vi "GetSRdata.vi"(8 "Error In":errorcluster) -> (0 "Error Out":errorcluster, 3 "SRList":T1 {"SR#" format="%#_10g"})   [LabVIEW 2017, in "Server.lvlib" / "Oracle.lvlib"]
uses:
  Oracle.lvlib
  TypeDefs/SR List.ctl
  TypeDefs/SR Data.ctl
  Server.lvlib
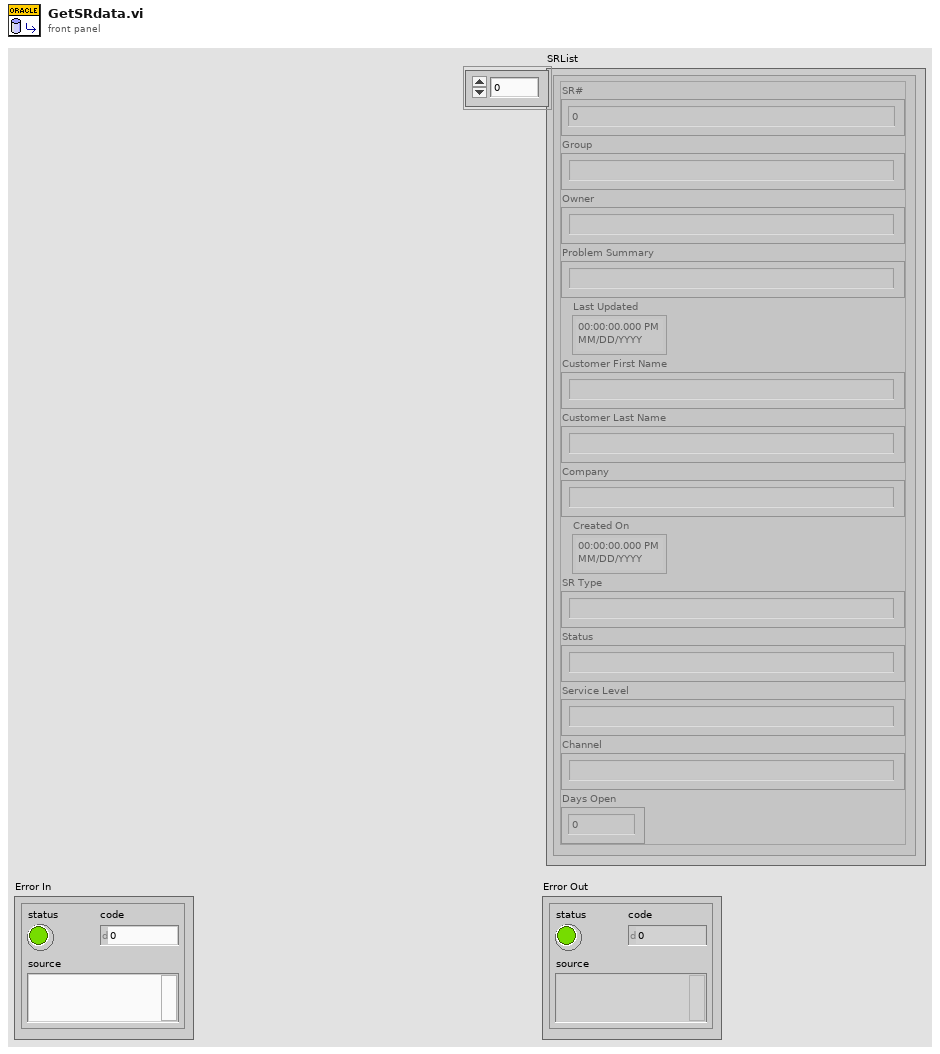
[diagram p1: front panel]
types:
  T1 = typedef "Server.lvlib/SR List.ctl" = T2[]
  T2 = typedef "Server.lvlib/SR Data.ctl" = cluster{"SR#":dbl, "Group":string, "Owner":string, "Problem Summary":string, "Last Updated":timestamp, "Customer First Name":string, "Customer Last Name":string, "Company":string, "Created On":timestamp, "SR Type":string, "Status":string, "Service Level":string, "Channel":string, "Days Open":dbl}
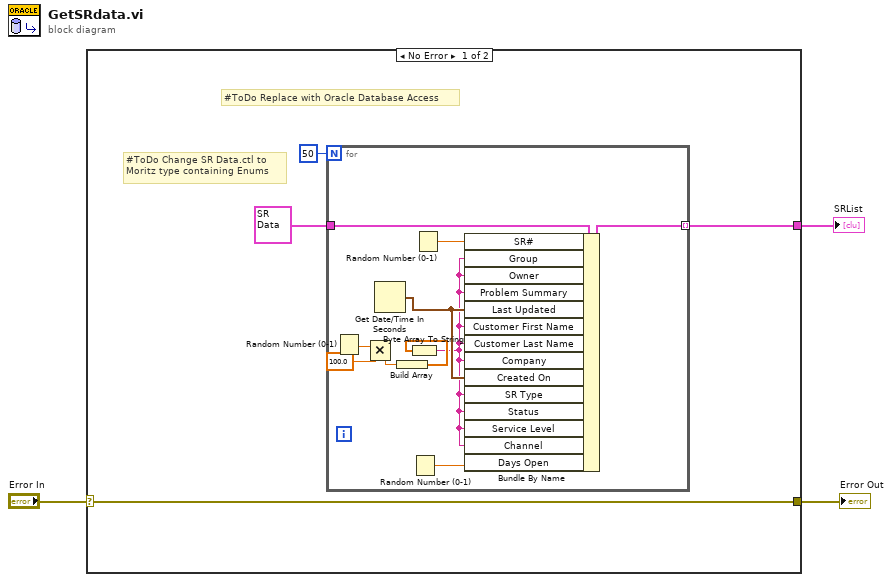
[diagram p0: block diagram]
diagram:
  n1 = case shown="No Error" "Error In" {
    selector: "Error In" -> [w7 w18]
    tunnel: [w7 w18] -> w2
    tunnel: [w5 _] -> w1
    frame No Error {
      # "#ToDo Change SR Data.ctl to\nMoritz type containing Enums"
      # "#ToDo Replace with Oracle Database Access"
      n2 = for {
        N: 50 -> [_]
        tunnel: T2 {"SR#"=0.0, "Group"="", "Owner"="", "Problem Summary"="", "Last Updated"=timestamp(0 s since 1904-01-01), "Customer First Name"="", "Customer Last Name"="", "Company"="", "Created On"=timestamp(0 s since 1904-01-01), "SR Type"="", "Status"="", "Service Level"="", "Channel"="", "Days Open"=0.0} ("SR Data") -> [w17]
        tunnel: [w16] -> w5 mode=indexing
        n3 = Random Number (0-1)() -> (number: 0 to 1=w13:dbl)
        n4 = Multiply(x=w13, y=100.0) -> (x*y=w11:dbl)
        n5 = Get Date/Time In Seconds() -> (seconds since 1Jan1904=w9:timestamp)
        n6 = Build Array(w11) -> (w10:dbl[])
        n7 = Byte Array To String(unsigned byte array=w10) -> (string=w8:string)
        n8 = Random Number (0-1)() -> (number: 0 to 1=w14:dbl)
        n9 = Random Number (0-1)() -> (number: 0 to 1=w15:dbl)
        n10 = Bundle By Name(cluster=w17, "SR#"=w15, "Group"=w8, "Owner"=w8, "Problem Summary"=w8, "Last Updated"=w9, "Customer First Name"=w8, "Customer Last Name"=w8, "Company"=w8, "Created On"=w9, "SR Type"=w8, "Status"=w8, "Service Level"=w8, "Channel"=w8, "Days Open"=w14) -> (w16:T2)
      }
    }
    frame Error {
    }
  }
  "Error Out" <- w2
  "SRList" <- w1
